vi "print graph.vi"(6 "channel strings":string[](array[string]), 8 "History Data":sgl[][](array[numeric]) format="%.2f", 9 "Y Scale Info":T2 {"Y Range"."Y Increment" format="%.2f"; "Y Range"."Y Maximum" format="%.2f"; "Y Range"."Y Minimum" format="%.2f"; "Yo and delta Y"."delta Y" format="%.2f"; "Yo and delta Y"."Yo" format="%.2f"}, 10 "X Scale Info":T1 {"X Range"."X Increment" format="%.2f"; "X Range"."X Maximum" format="%.2f"; "X Range"."X Minimum" format="%.2f"; "Xo and delta X"."delta X" format="%.2f"; "Xo and delta X"."Xo" format="%.2f"}, 11 "voltage chart":sgl[][](graph)) -> ()   [LabVIEW 2010]
panel:
  in  "?":bool
  # "Volts"
  # "time (s)"
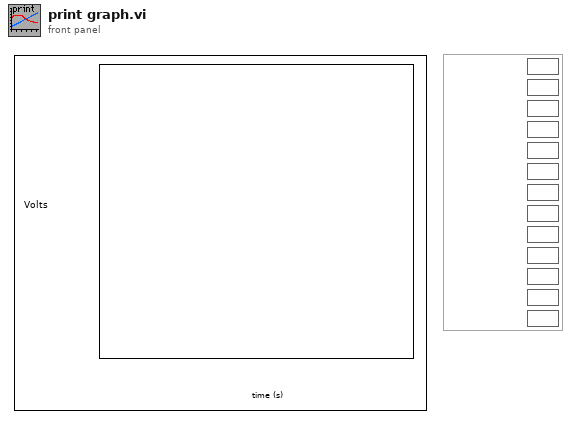
[diagram p1: front panel]
types:
  T1 = cluster{"X Scale Fit":u8, "Xo and delta X":cluster{"Xo":dbl, "delta X":dbl}, "X Style":u8, "X Format & Precision":cluster{"X Format":u8, "X Precision":u8}, "X Range":cluster{"X Minimum":dbl, "X Maximum":dbl, "X Increment":dbl}, "X Flipped":bool, "X Mapping Mode":u8, "X Editable":bool}
  T2 = cluster{"Y Scale Fit":u8, "Yo and delta Y":cluster{"Yo":dbl, "delta Y":dbl}, "Y Style":u8, "Y Format & Precision":cluster{"Y Format":u8, "Y Precision":u8}, "Y Range":cluster{"Y Minimum":dbl, "Y Maximum":dbl, "Y Increment":dbl}, "Y Flipped":bool, "Y Mapping Mode":u8, "Y Editable":bool}
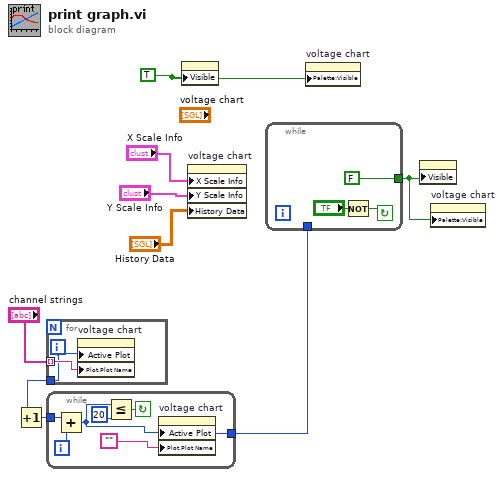
[diagram p0: block diagram]
diagram:
  w6 = TRUE
  n1 = for {
    tunnel: "channel strings" -> [w11] mode=indexing
    tunnel: [w10] -> w4
    i -> [w10]
    n2 = property on="voltage chart" class="WFChart (strict)"("Active Plot"=w10, "Plot.Plot Name"=w11) -> ()  [unwired: 2 in, 2 out]
  }
  n3 = Increment(x=w4) -> (x+1=w3:i32)
  n4 = while {
    tunnel: [w13] -> w1
    tunnel: w3 -> [w15]
    i -> [w14]
    stop <- w17 continue-if-true
    n5 = Add(x=w15, y=w14) -> (x+y=w13:i32)
    n6 = Less Or Equal?(x=w13, y=20) -> (x <= y?=w17:bool)
    n7 = property on="voltage chart" class="WFChart (strict)"("Active Plot"=w13, "Plot.Plot Name"="") -> ()  [unwired: 2 in, 2 out]
  }
  n8 = property class="Bool"("Visible"=w6) -> ()  [unwired: 2 in, 2 out]
  n9 = property on="voltage chart" class="WFChart (strict)"("X Scale Info"="X Scale Info", "Y Scale Info"="Y Scale Info", "History Data"="History Data") -> ()  [unwired: 2 in, 2 out]
  n10 = while {
    tunnel: w1 -> [_]
    tunnel: [FALSE] -> w5
    stop <- w19 continue-if-true
    n11 = Not(x="?") -> (.not. x?=w19:bool)
  }
  n12 = property on="voltage chart" class="WFChart (strict)"("Palette:Visible"=w6) -> ()  [unwired: 2 in, 2 out]
  n13 = property class="Bool"("Visible"=w5) -> ()  [unwired: 2 in, 2 out]
  n14 = property on="voltage chart" class="WFChart (strict)"("Palette:Visible"=w5) -> ()  [unwired: 2 in, 2 out]
